vi "Get Core Count.vi"(8 "error in (no error)":errorcluster, 11 "CPU Info in":refnum<class "CPU Info.lvclass">) -> (0 "error out":errorcluster, 2 "Core Count":i32, 3 "CPU Info out":refnum<class "CPU Info.lvclass">)   [LabVIEW 2017, in "DSF Core.lvlib" / "CPU Info.lvclass"]
uses:
  CPU Info.lvclass
  CPU Info.lvclass/CPU Info.ctl
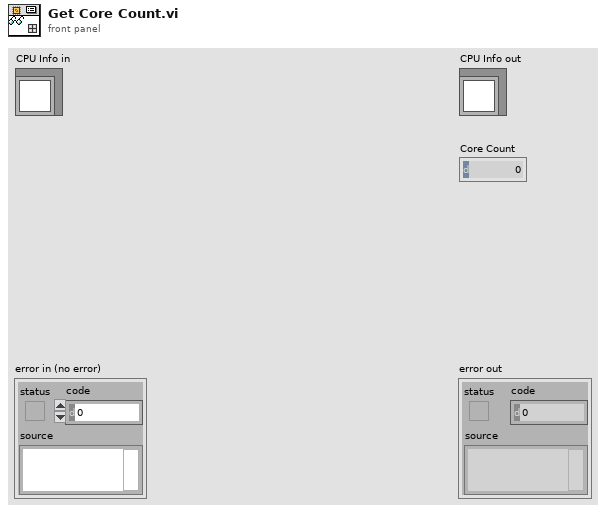
[diagram p1: front panel]
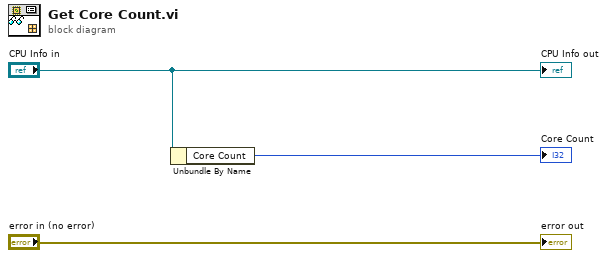
[diagram p0: block diagram]
diagram:
  n1 = Unbundle By Name("CPU Info in") -> ("Core Count"=→"Core Count":i32)
  "error out" <- "error in (no error)"
  "CPU Info out" <- "CPU Info in"
